vi "Get Query.vi"(8 "error in (no error)":errorcluster, 9 "HTML Entity (F)":bool, 11 "URI in":refnum<class "URI.lvclass">) -> (0 "error out":errorcluster, 2 "query":string, 3 "URI out":refnum<class "URI.lvclass">)   [LabVIEW 2013, in "openURI.lvlib" / "URI.lvclass"]
uses:
  URI.lvclass
  URI.lvclass/URI.ctl
  components/query/URI-Component.Query.lvclass
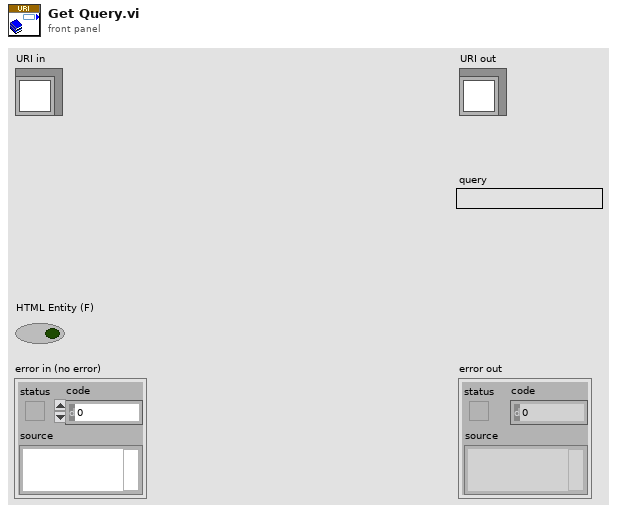
[diagram p1: front panel]
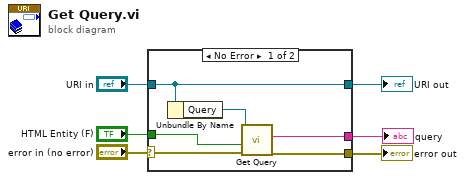
[diagram p0: block diagram]
diagram:
  n1 = case shown="No Error" "error in (no error)" {
    selector: "error in (no error)" -> [w11 w14]
    tunnel: [w10 w14] -> w5
    tunnel: [w9 w13] -> w3
    tunnel: "URI in" -> [w9 w13]
    tunnel: [w12 _] -> w2
    tunnel: "HTML Entity (F)" -> [w7 _]
    frame No Error {
      n2 = Unbundle By Name(w9) -> ("Query"=w8:refnum<class "URI-Component.Query.lvclass">)
      n3 = call "Get Query.vi"("error in (no error)"=w11, "HTML Entity (F)"=w7, "URI-Component.Path in"=w8) -> ("error out"=w10:errorcluster, "query-component"=w12:string)  [unwired: 6 in, 1 out]
    }
    frame Error {
    }
  }
  "error out" <- w5
  "URI out" <- w3
  "query" <- w2
